vi "McP-Dbl2String v0.3.vi"(1 "McP Input Number":dbl=72356.0 format="%.1f") -> (0 "Controller String":string="+72356\r")   [LabVIEW 2021]
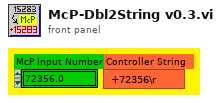
[diagram p1: front panel]
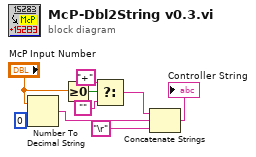
[diagram p0: block diagram]
diagram:
  n1 = Number To Decimal String(number="McP Input Number", width (-)=0) -> (decimal integer string=w3:string)
  n2 = Greater Or Equal To 0?(x="McP Input Number") -> (x >= 0?=w5:bool)
  n3 = Select(t="+", s=w5, f="") -> (s? t:f=w8:string)
  n4 = Concatenate Strings(w8, w3, "\r") -> (→"Controller String":string)
